vi "Select work order from drop down.vi"(8 "error in (no error)":errorcluster) -> (0 "error out":errorcluster, 2 "Work order info":string, 3 "work order":string)   [LabVIEW 2013]
panel:
  in  "Work Order (pick from drop down list)":u16(ring) items=["Select work order", "WO41792, PN=F-SYN-1000330-1G, Qty=300", "WO40930, PN=F-SYN-1000336-1G, Qty=100", "WO40717, PN=F-SYN-1000334G, Qty=288"]
  in  "Work order list":string[](array[string])
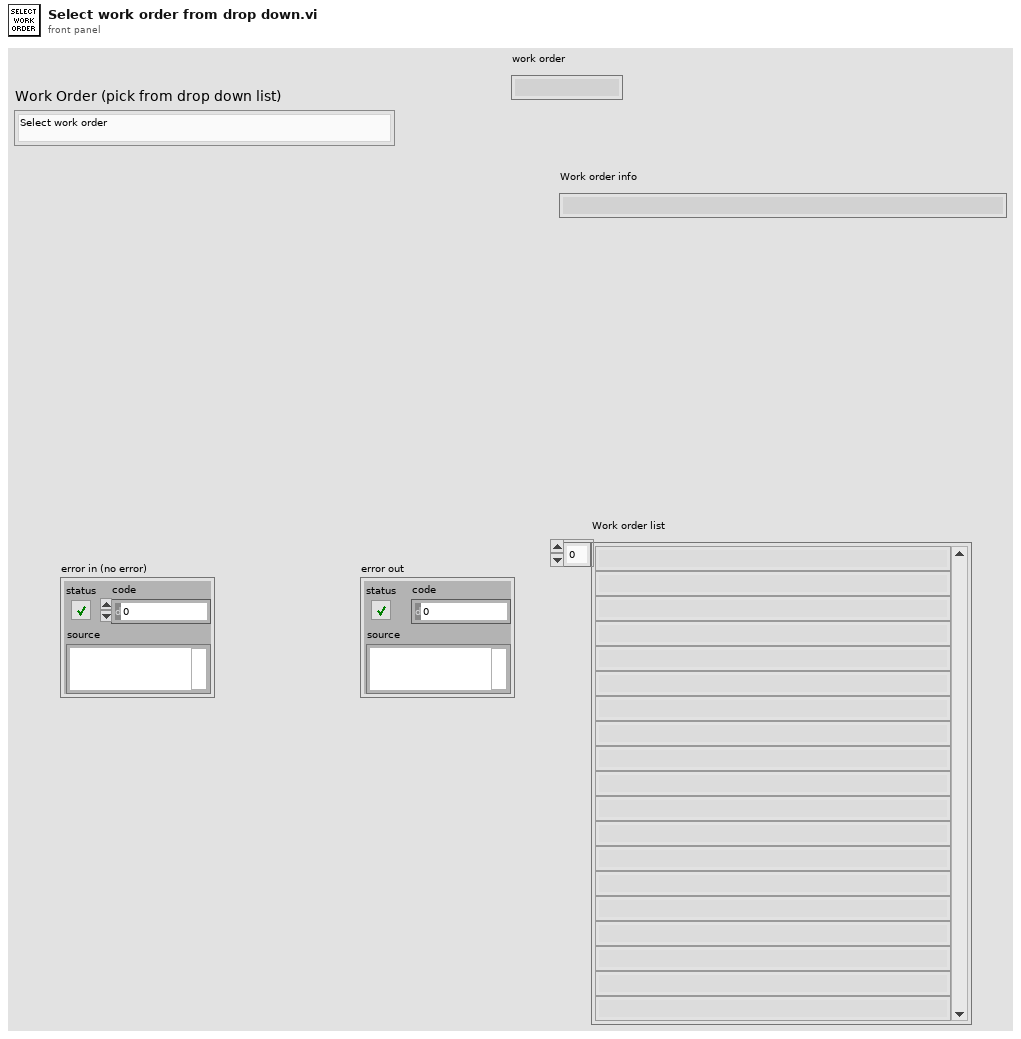
[diagram p1: front panel]
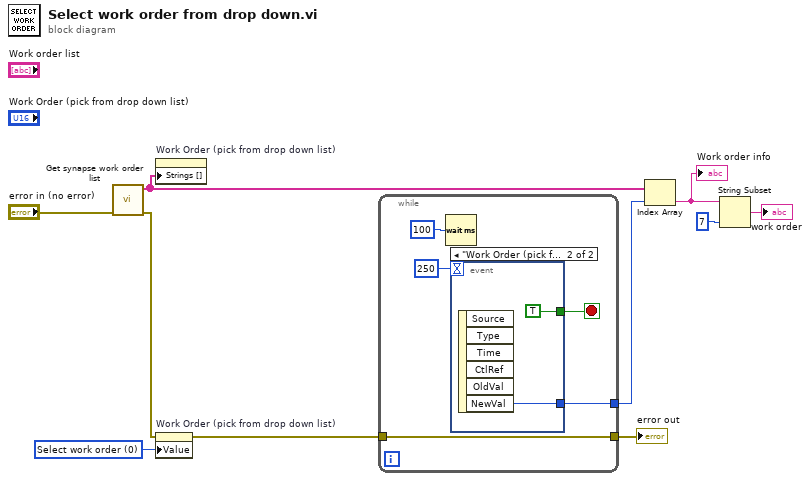
[diagram p0: block diagram]
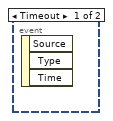
[diagram p2: hidden frame]
diagram:
  w1 = u16 0 items=["Select work order", "WO41792, PN=F-SYN-1000330-1G, Qty=300", "WO40930, PN=F-SYN-1000336-1G, Qty=100", "WO40717, PN=F-SYN-1000334G, Qty=288"] ("Work Order (pick from drop down list)")
  n1 = call "Get synapse work order list.vi"("error in (no error)"="error in (no error)") -> ("error out"=w3:errorcluster, "Work order list"=w8:string[])  [unwired: 9 in]
  n2 = property on="Work Order (pick from drop down list)" class="Ring (strict)"("Strings []"=w8) -> ()  [unwired: 2 in, 2 out]
  n3 = property on="Work Order (pick from drop down list)" class="Ring (strict)"(error in=w3, "Value"=w1) -> (error out=w2:errorcluster)  [unwired: 1 in, 1 out]
  n4 = while {
    tunnel: [w15] -> w9
    tunnel: w2 -> [w15]
    tunnel: [w13] -> w7
    stop <- w14 stop-if-true
    n5 = Wait (ms)(milliseconds to wait=u32 100) -> ()  [unwired: 1 out]
    n6 = event shown="[1] \"Work Order (pick from drop down list)\": Value Change" {
      selector: _ -> [_ _]
      dyn-events: _ -> [_ _]
      timeout: 250 -> [_ _]
      tunnel: [_ TRUE] -> w14
      tunnel: [_ w16] -> w13
      event Timeout {
        n7 = event-data() -> ()  [unwired: 1 in, 3 out]
      }
      event "Work Order (pick from drop down list)": Value Change {
        n8 = event-data() -> ("NewVal"=w16:u16)  [unwired: 1 in, 5 out]
      }
    }
  }
  "error out" <- w9
  n9 = Index Array(array=w8, index=w7) -> (element=w6:string)
  "Work order info" <- w6
  n10 = String Subset(string=w6, length (rest)=7 ("length (rest)")) -> (substring=→"work order":string)  [unwired: 1 in]
